vi "Joystick control (SubVI).vi"() -> (0 "Boolean 6":bool, 1 "Boolean 8":bool, 2 "Boolean 7":bool, 3 "Boolean 5":bool, 4 "Boolean 2":bool, 5 "Boolean":bool, 6 "Boolean 3":bool, 7 "Boolean 4":bool)   [LabVIEW 2017]
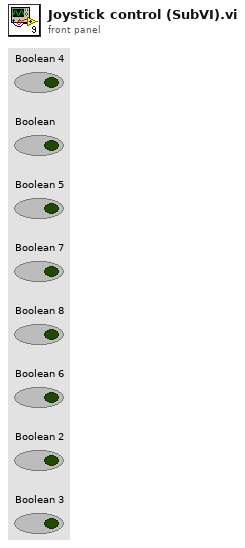
[diagram p1: front panel]
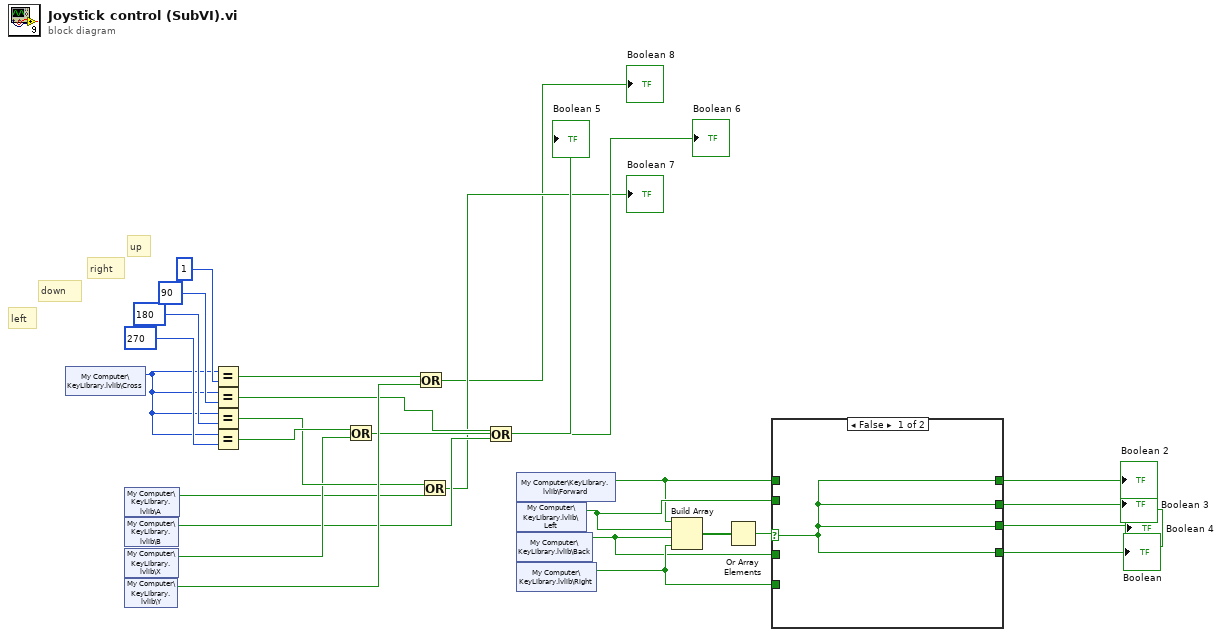
[diagram p0: block diagram]
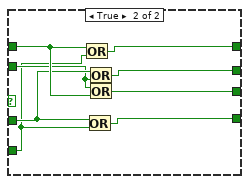
[diagram p2: hidden frame]
diagram:
  # "left"
  # "down"
  # "right"
  # "up"
  n1 = shared-variable "My Computer\\KeyLibrary.lvlib\\Cross"() -> (w1:i32)  [unwired: 1 in, 1 out]
  n2 = shared-variable "My Computer\\KeyLibrary.lvlib\\A"() -> (w6:bool)  [unwired: 1 in, 1 out]
  n3 = shared-variable "My Computer\\KeyLibrary.lvlib\\B"() -> (w7:bool)  [unwired: 1 in, 1 out]
  n4 = shared-variable "My Computer\\KeyLibrary.lvlib\\X"() -> (w8:bool)  [unwired: 1 in, 1 out]
  n5 = shared-variable "My Computer\\KeyLibrary.lvlib\\Y"() -> (w17:bool)  [unwired: 1 in, 1 out]
  n6 = Equal?(x=w1, y=1) -> (x = y?=w13:bool)
  n7 = Equal?(x=w1, y=90) -> (x = y?=w14:bool)
  n8 = Equal?(x=w1, y=180) -> (x = y?=w15:bool)
  n9 = Equal?(x=w1, y=270) -> (x = y?=w16:bool)
  n10 = Or(x=w16, y=w8) -> (x .or. y?=→"Boolean 5":bool)
  n11 = Or(x=w13, y=w17) -> (x .or. y?=→"Boolean 8":bool)
  n12 = Or(x=w15, y=w6) -> (x .or. y?=→"Boolean 7":bool)
  n13 = Or(x=w14, y=w7) -> (x .or. y?=→"Boolean 6":bool)
  n14 = shared-variable "My Computer\\KeyLibrary.lvlib\\Forward"() -> (w20:bool)  [unwired: 1 in, 1 out]
  n15 = shared-variable "My Computer\\KeyLibrary.lvlib\\Left"() -> (w22:bool)  [unwired: 1 in, 1 out]
  n16 = shared-variable "My Computer\\KeyLibrary.lvlib\\Back"() -> (w21:bool)  [unwired: 1 in, 1 out]
  n17 = shared-variable "My Computer\\KeyLibrary.lvlib\\Right"() -> (w23:bool)  [unwired: 1 in, 1 out]
  n18 = Build Array(w20, w22, w21, w23) -> (w19:bool[])
  n19 = Or Array Elements(Boolean array=w19) -> (logical OR=w18:bool)
  n20 = case shown="False" w18 {
    selector: w18 -> [w28 _]
    tunnel: w20 -> [_ w36]
    tunnel: w21 -> [_ w35]
    tunnel: w22 -> [_ w34]
    tunnel: w23 -> [_ w33]
    tunnel: [w28 w32] -> w24
    tunnel: [w28 w31] -> w25
    tunnel: [w28 w30] -> w26
    tunnel: [w28 w29] -> w27
    frame False {
    }
    frame True {
      n21 = Or(x=w36, y=w33) -> (x .or. y?=w30:bool)
      n22 = Or(x=w35, y=w33) -> (x .or. y?=w29:bool)
      n23 = Or(x=w35, y=w34) -> (x .or. y?=w31:bool)
      n24 = Or(x=w34, y=w36) -> (x .or. y?=w32:bool)
    }
  }
  "Boolean" <- w27
  "Boolean 2" <- w26
  "Boolean 3" <- w25
  "Boolean 4" <- w24
